vi "flow-percent-volume-flow.vi"(8 "Measure Percentage":dbl, 10 "Sensor Max Percentage":dbl=100.42, 11 "Sensor Max Flow":dbl=502.08) -> (0 "volumetric flow (ml/min)":dbl)   [LabVIEW 2023]
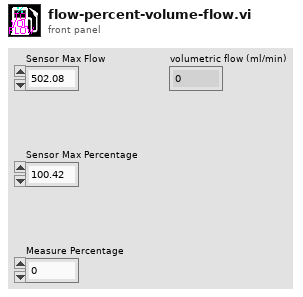
[diagram p1: front panel]
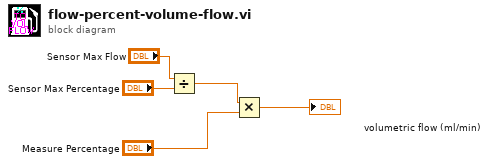
[diagram p0: block diagram]
diagram:
  n1 = Divide(x="Sensor Max Flow", y="Sensor Max Percentage") -> (x/y=w2:dbl)
  n2 = Multiply(x=w2, y="Measure Percentage") -> (x*y=→"volumetric flow (ml/min)":dbl)
